vi "Field vs  IV and Ic distribution_V3.vi"() -> ()   [LabVIEW 2021]
uses:
  RT fast data.ctl
  <vilib>/LabVIEW Targets/FPGA/cRIO/shared/nicrio_ModuleControls/nicrio_cRIO-9775_RecordDataRates4ChansRing.ctl
  <vilib>/Utility/file.llb/Write Delimited Spreadsheet (DBL).vi
  Transport measurement/VIs/global.vi
  <resource>/objmgr/ni.dex.rc
  <vilib>/Analysis/NI_AALBase.lvlib
panel:
  in  "Tab Control":enum32{"Field", "cRIO", "IV Ic Parameters"}(tab)
  in  "Field Rate mT per sec":dbl=0.1 format="%#_13g"
  in  "Field Radius mT":dbl=12.0 format="%#_13g"
  in  "Field step mT":dbl=0.05 format="%#_13g"
  in  "Field Origin mT":dbl=-6.0 format="%#_13g"
  in  "Ramp up first T":bool=TRUE
  in  "Ramp type":string(combo)="Range"
  in  "Field Device Select":string(combo)="Elsa Magnet mT"
  in  "Power dbm":dbl=-135.0 format="%#_13g"
  in  "Field sub select":string(combo)="50mApV"
  in  "AI Channel":u8
  in  "Trigger Slope":enum8{"Positive", "Negative"}(ring)
  in  "Dist Record Samples":u32=10000
  in  "cRIO IP":string="//172.22.11.2"
  in  "Data buffer size":i32=1000
  in  "Voltage Scale factor":dbl=0.0001
  in  "Current Scale factor":dbl=1.0
  in  "IV Record Samples":u32=5000
  in  "Gate wait time us":u32=150
  in  "IV Record Data Rate":T1=200 items=["20.000 MS/s (NI 9775)"=1, "10.00 MS/s (NI 9775)"=2, "6.667 MS/s (NI 9775)"=3, "5.000 MS/s (NI 9775)"=4, "2.500 MS/s (NI 9775)"=8, "1.667 MS/s (NI 9775)"=12, "1.250 MS/s (NI 9775)"=16, "1.000 MS/s (NI 9775)"=20, "833.333 KS/s (NI 9775)"=24, "714.286 KS/s (NI 9775)"=28, "625.000 KS/s (NI 9775)"=32, "555.556 KS/s (NI 9775)"=36, "500.000 KS/s (NI 9775)"=40, "454.545 KS/s (NI 9775)"=44, "416.667 KS/s (NI 9775)"=48, "384.615 KS/s (NI 9775)"=52, "357.143 KS/s (NI 9775)"=56, "333.333 KS/s (NI 9775)"=60, "312.500 KS/s (NI 9775)"=64, "294.118 KS/s (NI 9775)"=68, "277.778 KS/s (NI 9775)"=72, "263.158 KS/s (NI 9775)"=76, "250.000 KS/s (NI 9775)"=80, "238.095 KS/s (NI 9775)"=84, "227.273 KS/s (NI 9775)"=88, "217.391 KS/s (NI 9775)"=92, "208.333 KS/s (NI 9775)"=96, "200.000 KS/s (NI 9775)"=100, "192.308 KS/s (NI 9775)"=104, "185.185 KS/s (NI 9775)"=108, "178.571 KS/s (NI 9775)"=112, "172.414 KS/s (NI 9775)"=116, "166.667 KS/s (NI 9775)"=120, "161.290 KS/s (NI 9775)"=124, "156.250 KS/s (NI 9775)"=128, "151.515 KS/s (NI 9775)"=132, "147.059 KS/s (NI 9775)"=136, "142.857 KS/s (NI 9775)"=140, "138.889 KS/s (NI 9775)"=144, "135.135 KS/s (NI 9775)"=148, "131.579 KS/s (NI 9775)"=152, "128.205 KS/s (NI 9775)"=156, "125.000 KS/s (NI 9775)"=160, "121.951 KS/s (NI 9775)"=164, "119.048 KS/s (NI 9775)"=168, "116.279 KS/s (NI 9775)"=172, "113.636 KS/s (NI 9775)"=176, "111.111 KS/s (NI 9775)"=180, "108.696 KS/s (NI 9775)"=184, "106.383 KS/s (NI 9775)"=188, "104.167 KS/s (NI 9775)"=192, "102.041 KS/s (NI 9775)"=196, "100.000 KS/s (NI 9775)"=200, "50.000 KS/s (NI 9775)"=400, "33.333 KS/s (NI 9775)"=600, "25.000 KS/s (NI 9775)"=800, "20.000 KS/s (NI 9775)"=1000, "16.667 KS/s (NI 9775)"=1200, "14.286 KS/s (NI 9775)"=1400, "12.500 KS/s (NI 9775)"=1600, "11.111 KS/s (NI 9775)"=1800, "10.000 KS/s (NI 9775)"=2000, "9.091 KS/s (NI 9775)"=2200, "8.333 KS/s (NI 9775)"=2400, "7.692 KS/s (NI 9775)"=2600, "7.143 KS/s (NI 9775)"=2800, "6.667 KS/s (NI 9775)"=3000, "6.250 KS/s (NI 9775)"=3200, "5.882 KS/s (NI 9775)"=3400, "5.556 KS/s (NI 9775)"=3600, "5.000 KS/s (NI 9775)"=4000, "4.762 KS/s (NI 9775)"=4200, "4.545 KS/s (NI 9775)"=4400, "4.348 KS/s (NI 9775)"=4600, "4.167 KS/s (NI 9775)"=4800, "4.000 KS/s (NI 9775)"=5000, "3.846 KS/s (NI 9775)"=5200, "3.571 KS/s (NI 9775)"=5600, "3.333 KS/s (NI 9775)"=6000, "3.125 KS/s (NI 9775)"=6400, "2.941 KS/s (NI 9775)"=6800, "2.778 KS/s (NI 9775)"=7200, "2.632 KS/s (NI 9775)"=7600, "2.500 KS/s (NI 9775)"=8000, "2.381 KS/s (NI 9775)"=8400, "2.273 KS/s (NI 9775)"=8800, "2.174 KS/s (NI 9775)"=9200, "2.083 KS/s (NI 9775)"=9600, "2.000 KS/s (NI 9775)"=10000, "1.923 KS/s (NI 9775)"=10400, "1.852 KS/s (NI 9775)"=10800, "1.786 KS/s (NI 9775)"=11200, "1.724 KS/s (NI 9775)"=11600, "1.667 KS/s (NI 9775)"=12000, "1.613 KS/s (NI 9775)"=12400, "1.563 KS/s (NI 9775)"=12800, "1.515 KS/s (NI 9775)"=13200, "1.471 KS/s (NI 9775)"=13600, "1.429 KS/s (NI 9775)"=14000, "1.389 KS/s (NI 9775)"=14400, "1.351 KS/s (NI 9775)"=14800, "1.316 KS/s (NI 9775)"=15200, "1.282 KS/s (NI 9775)"=15600, "1.250 KS/s (NI 9775)"=16000, "1.220 KS/s (NI 9775)"=16400, "1.190 KS/s (NI 9775)"=16800, "1.163 KS/s (NI 9775)"=17200, "1.136 KS/s (NI 9775)"=17600, "1.111 KS/s (NI 9775)"=18000, "1.087 KS/s (NI 9775)"=18400, "1.064 KS/s (NI 9775)"=18800, "1.042 KS/s (NI 9775)"=19200, "1.020 KS/s (NI 9775)"=19600, "1.000 KS/s (NI 9775)"=20000, "0.980 KS/s (NI 9775)"=20400, "0.962 KS/s (NI 9775)"=20800, "0.943 KS/s (NI 9775)"=21200, "0.926 KS/s (NI 9775)"=21600, "0.909 KS/s (NI 9775)"=22000, "0.893 KS/s (NI 9775)"=22400, "0.877 KS/s (NI 9775)"=22800, "0.862 KS/s (NI 9775)"=23200, "0.847 KS/s (NI 9775)"=23600, "0.833 KS/s (NI 9775)"=24000, "0.820 KS/s (NI 9775)"=24400, "0.806 KS/s (NI 9775)"=24800, "0.794 KS/s (NI 9775)"=25200, "0.781 KS/s (NI 9775)"=25600, "0.694 KS/s (NI 9775)"=28800, "0.625 KS/s (NI 9775)"=32000, "0.568 KS/s (NI 9775)"=35200, "0.521 KS/s (NI 9775)"=38400, "0.446 KS/s (NI 9775)"=44800, "0.391 KS/s (NI 9775)"=51200, "0.347 KS/s (NI 9775)"=57600, "0.313 KS/s (NI 9775)"=64000]
  in  "Relative threshold":dbl=0.25 format="%#_13g"
  in  "Dist Record Data Rate":T1=1 items=["20.000 MS/s (NI 9775)"=1, "10.00 MS/s (NI 9775)"=2, "6.667 MS/s (NI 9775)"=3, "5.000 MS/s (NI 9775)"=4, "2.500 MS/s (NI 9775)"=8, "1.667 MS/s (NI 9775)"=12, "1.250 MS/s (NI 9775)"=16, "1.000 MS/s (NI 9775)"=20, "833.333 KS/s (NI 9775)"=24, "714.286 KS/s (NI 9775)"=28, "625.000 KS/s (NI 9775)"=32, "555.556 KS/s (NI 9775)"=36, "500.000 KS/s (NI 9775)"=40, "454.545 KS/s (NI 9775)"=44, "416.667 KS/s (NI 9775)"=48, "384.615 KS/s (NI 9775)"=52, "357.143 KS/s (NI 9775)"=56, "333.333 KS/s (NI 9775)"=60, "312.500 KS/s (NI 9775)"=64, "294.118 KS/s (NI 9775)"=68, "277.778 KS/s (NI 9775)"=72, "263.158 KS/s (NI 9775)"=76, "250.000 KS/s (NI 9775)"=80, "238.095 KS/s (NI 9775)"=84, "227.273 KS/s (NI 9775)"=88, "217.391 KS/s (NI 9775)"=92, "208.333 KS/s (NI 9775)"=96, "200.000 KS/s (NI 9775)"=100, "192.308 KS/s (NI 9775)"=104, "185.185 KS/s (NI 9775)"=108, "178.571 KS/s (NI 9775)"=112, "172.414 KS/s (NI 9775)"=116, "166.667 KS/s (NI 9775)"=120, "161.290 KS/s (NI 9775)"=124, "156.250 KS/s (NI 9775)"=128, "151.515 KS/s (NI 9775)"=132, "147.059 KS/s (NI 9775)"=136, "142.857 KS/s (NI 9775)"=140, "138.889 KS/s (NI 9775)"=144, "135.135 KS/s (NI 9775)"=148, "131.579 KS/s (NI 9775)"=152, "128.205 KS/s (NI 9775)"=156, "125.000 KS/s (NI 9775)"=160, "121.951 KS/s (NI 9775)"=164, "119.048 KS/s (NI 9775)"=168, "116.279 KS/s (NI 9775)"=172, "113.636 KS/s (NI 9775)"=176, "111.111 KS/s (NI 9775)"=180, "108.696 KS/s (NI 9775)"=184, "106.383 KS/s (NI 9775)"=188, "104.167 KS/s (NI 9775)"=192, "102.041 KS/s (NI 9775)"=196, "100.000 KS/s (NI 9775)"=200, "50.000 KS/s (NI 9775)"=400, "33.333 KS/s (NI 9775)"=600, "25.000 KS/s (NI 9775)"=800, "20.000 KS/s (NI 9775)"=1000, "16.667 KS/s (NI 9775)"=1200, "14.286 KS/s (NI 9775)"=1400, "12.500 KS/s (NI 9775)"=1600, "11.111 KS/s (NI 9775)"=1800, "10.000 KS/s (NI 9775)"=2000, "9.091 KS/s (NI 9775)"=2200, "8.333 KS/s (NI 9775)"=2400, "7.692 KS/s (NI 9775)"=2600, "7.143 KS/s (NI 9775)"=2800, "6.667 KS/s (NI 9775)"=3000, "6.250 KS/s (NI 9775)"=3200, "5.882 KS/s (NI 9775)"=3400, "5.556 KS/s (NI 9775)"=3600, "5.000 KS/s (NI 9775)"=4000, "4.762 KS/s (NI 9775)"=4200, "4.545 KS/s (NI 9775)"=4400, "4.348 KS/s (NI 9775)"=4600, "4.167 KS/s (NI 9775)"=4800, "4.000 KS/s (NI 9775)"=5000, "3.846 KS/s (NI 9775)"=5200, "3.571 KS/s (NI 9775)"=5600, "3.333 KS/s (NI 9775)"=6000, "3.125 KS/s (NI 9775)"=6400, "2.941 KS/s (NI 9775)"=6800, "2.778 KS/s (NI 9775)"=7200, "2.632 KS/s (NI 9775)"=7600, "2.500 KS/s (NI 9775)"=8000, "2.381 KS/s (NI 9775)"=8400, "2.273 KS/s (NI 9775)"=8800, "2.174 KS/s (NI 9775)"=9200, "2.083 KS/s (NI 9775)"=9600, "2.000 KS/s (NI 9775)"=10000, "1.923 KS/s (NI 9775)"=10400, "1.852 KS/s (NI 9775)"=10800, "1.786 KS/s (NI 9775)"=11200, "1.724 KS/s (NI 9775)"=11600, "1.667 KS/s (NI 9775)"=12000, "1.613 KS/s (NI 9775)"=12400, "1.563 KS/s (NI 9775)"=12800, "1.515 KS/s (NI 9775)"=13200, "1.471 KS/s (NI 9775)"=13600, "1.429 KS/s (NI 9775)"=14000, "1.389 KS/s (NI 9775)"=14400, "1.351 KS/s (NI 9775)"=14800, "1.316 KS/s (NI 9775)"=15200, "1.282 KS/s (NI 9775)"=15600, "1.250 KS/s (NI 9775)"=16000, "1.220 KS/s (NI 9775)"=16400, "1.190 KS/s (NI 9775)"=16800, "1.163 KS/s (NI 9775)"=17200, "1.136 KS/s (NI 9775)"=17600, "1.111 KS/s (NI 9775)"=18000, "1.087 KS/s (NI 9775)"=18400, "1.064 KS/s (NI 9775)"=18800, "1.042 KS/s (NI 9775)"=19200, "1.020 KS/s (NI 9775)"=19600, "1.000 KS/s (NI 9775)"=20000, "0.980 KS/s (NI 9775)"=20400, "0.962 KS/s (NI 9775)"=20800, "0.943 KS/s (NI 9775)"=21200, "0.926 KS/s (NI 9775)"=21600, "0.909 KS/s (NI 9775)"=22000, "0.893 KS/s (NI 9775)"=22400, "0.877 KS/s (NI 9775)"=22800, "0.862 KS/s (NI 9775)"=23200, "0.847 KS/s (NI 9775)"=23600, "0.833 KS/s (NI 9775)"=24000, "0.820 KS/s (NI 9775)"=24400, "0.806 KS/s (NI 9775)"=24800, "0.794 KS/s (NI 9775)"=25200, "0.781 KS/s (NI 9775)"=25600, "0.694 KS/s (NI 9775)"=28800, "0.625 KS/s (NI 9775)"=32000, "0.568 KS/s (NI 9775)"=35200, "0.521 KS/s (NI 9775)"=38400, "0.446 KS/s (NI 9775)"=44800, "0.391 KS/s (NI 9775)"=51200, "0.347 KS/s (NI 9775)"=57600, "0.313 KS/s (NI 9775)"=64000]
  in  "Zero avg":i32=500
  in  "Count us half of T":u32=1
  in  "Wait before trigger us":u32=10100
  in  "Tab Control 2":enum32{"IV", "Ic"}(tab)
  out "IV parameters":T2={"Records Num"=1, "AI Trigger Configuration"={"Trigger Slope"=enum."Positive", "Trigger Level"=0.10009765625, "Hystesis Value"=0.094970703125, "AI Channel"=0}, "Record PreTrigger Samples"=1, "Record Samples"=5000, "Ic Cut off or curve"=FALSE, "Gate wait time us"=150, "Record Data Rate"=200, "Count us half of T"=1, "Wait before trigger us"=10100, "Cutoff delay usec"=0} {"Record Data Rate" items=["20.000 MS/s (NI 9775)"=1, "10.00 MS/s (NI 9775)"=2, "6.667 MS/s (NI 9775)"=3, "5.000 MS/s (NI 9775)"=4, "2.500 MS/s (NI 9775)"=8, "1.667 MS/s (NI 9775)"=12, "1.250 MS/s (NI 9775)"=16, "1.000 MS/s (NI 9775)"=20, "833.333 KS/s (NI 9775)"=24, "714.286 KS/s (NI 9775)"=28, "625.000 KS/s (NI 9775)"=32, "555.556 KS/s (NI 9775)"=36, "500.000 KS/s (NI 9775)"=40, "454.545 KS/s (NI 9775)"=44, "416.667 KS/s (NI 9775)"=48, "384.615 KS/s (NI 9775)"=52, "357.143 KS/s (NI 9775)"=56, "333.333 KS/s (NI 9775)"=60, "312.500 KS/s (NI 9775)"=64, "294.118 KS/s (NI 9775)"=68, "277.778 KS/s (NI 9775)"=72, "263.158 KS/s (NI 9775)"=76, "250.000 KS/s (NI 9775)"=80, "238.095 KS/s (NI 9775)"=84, "227.273 KS/s (NI 9775)"=88, "217.391 KS/s (NI 9775)"=92, "208.333 KS/s (NI 9775)"=96, "200.000 KS/s (NI 9775)"=100, "192.308 KS/s (NI 9775)"=104, "185.185 KS/s (NI 9775)"=108, "178.571 KS/s (NI 9775)"=112, "172.414 KS/s (NI 9775)"=116, "166.667 KS/s (NI 9775)"=120, "161.290 KS/s (NI 9775)"=124, "156.250 KS/s (NI 9775)"=128, "151.515 KS/s (NI 9775)"=132, "147.059 KS/s (NI 9775)"=136, "142.857 KS/s (NI 9775)"=140, "138.889 KS/s (NI 9775)"=144, "135.135 KS/s (NI 9775)"=148, "131.579 KS/s (NI 9775)"=152, "128.205 KS/s (NI 9775)"=156, "125.000 KS/s (NI 9775)"=160, "121.951 KS/s (NI 9775)"=164, "119.048 KS/s (NI 9775)"=168, "116.279 KS/s (NI 9775)"=172, "113.636 KS/s (NI 9775)"=176, "111.111 KS/s (NI 9775)"=180, "108.696 KS/s (NI 9775)"=184, "106.383 KS/s (NI 9775)"=188, "104.167 KS/s (NI 9775)"=192, "102.041 KS/s (NI 9775)"=196, "100.000 KS/s (NI 9775)"=200, "50.000 KS/s (NI 9775)"=400, "33.333 KS/s (NI 9775)"=600, "25.000 KS/s (NI 9775)"=800, "20.000 KS/s (NI 9775)"=1000, "16.667 KS/s (NI 9775)"=1200, "14.286 KS/s (NI 9775)"=1400, "12.500 KS/s (NI 9775)"=1600, "11.111 KS/s (NI 9775)"=1800, "10.000 KS/s (NI 9775)"=2000, "9.091 KS/s (NI 9775)"=2200, "8.333 KS/s (NI 9775)"=2400, "7.692 KS/s (NI 9775)"=2600, "7.143 KS/s (NI 9775)"=2800, "6.667 KS/s (NI 9775)"=3000, "6.250 KS/s (NI 9775)"=3200, "5.882 KS/s (NI 9775)"=3400, "5.556 KS/s (NI 9775)"=3600, "5.000 KS/s (NI 9775)"=4000, "4.762 KS/s (NI 9775)"=4200, "4.545 KS/s (NI 9775)"=4400, "4.348 KS/s (NI 9775)"=4600, "4.167 KS/s (NI 9775)"=4800, "4.000 KS/s (NI 9775)"=5000, "3.846 KS/s (NI 9775)"=5200, "3.571 KS/s (NI 9775)"=5600, "3.333 KS/s (NI 9775)"=6000, "3.125 KS/s (NI 9775)"=6400, "2.941 KS/s (NI 9775)"=6800, "2.778 KS/s (NI 9775)"=7200, "2.632 KS/s (NI 9775)"=7600, "2.500 KS/s (NI 9775)"=8000, "2.381 KS/s (NI 9775)"=8400, "2.273 KS/s (NI 9775)"=8800, "2.174 KS/s (NI 9775)"=9200, "2.083 KS/s (NI 9775)"=9600, "2.000 KS/s (NI 9775)"=10000, "1.923 KS/s (NI 9775)"=10400, "1.852 KS/s (NI 9775)"=10800, "1.786 KS/s (NI 9775)"=11200, "1.724 KS/s (NI 9775)"=11600, "1.667 KS/s (NI 9775)"=12000, "1.613 KS/s (NI 9775)"=12400, "1.563 KS/s (NI 9775)"=12800, "1.515 KS/s (NI 9775)"=13200, "1.471 KS/s (NI 9775)"=13600, "1.429 KS/s (NI 9775)"=14000, "1.389 KS/s (NI 9775)"=14400, "1.351 KS/s (NI 9775)"=14800, "1.316 KS/s (NI 9775)"=15200, "1.282 KS/s (NI 9775)"=15600, "1.250 KS/s (NI 9775)"=16000, "1.220 KS/s (NI 9775)"=16400, "1.190 KS/s (NI 9775)"=16800, "1.163 KS/s (NI 9775)"=17200, "1.136 KS/s (NI 9775)"=17600, "1.111 KS/s (NI 9775)"=18000, "1.087 KS/s (NI 9775)"=18400, "1.064 KS/s (NI 9775)"=18800, "1.042 KS/s (NI 9775)"=19200, "1.020 KS/s (NI 9775)"=19600, "1.000 KS/s (NI 9775)"=20000, "0.980 KS/s (NI 9775)"=20400, "0.962 KS/s (NI 9775)"=20800, "0.943 KS/s (NI 9775)"=21200, "0.926 KS/s (NI 9775)"=21600, "0.909 KS/s (NI 9775)"=22000, "0.893 KS/s (NI 9775)"=22400, "0.877 KS/s (NI 9775)"=22800, "0.862 KS/s (NI 9775)"=23200, "0.847 KS/s (NI 9775)"=23600, "0.833 KS/s (NI 9775)"=24000, "0.820 KS/s (NI 9775)"=24400, "0.806 KS/s (NI 9775)"=24800, "0.794 KS/s (NI 9775)"=25200, "0.781 KS/s (NI 9775)"=25600, "0.694 KS/s (NI 9775)"=28800, "0.625 KS/s (NI 9775)"=32000, "0.568 KS/s (NI 9775)"=35200, "0.521 KS/s (NI 9775)"=38400, "0.446 KS/s (NI 9775)"=44800, "0.391 KS/s (NI 9775)"=51200, "0.347 KS/s (NI 9775)"=57600, "0.313 KS/s (NI 9775)"=64000]}
  out "Ic parameters":T2={"Records Num"=10000, "AI Trigger Configuration"={"Trigger Slope"=enum."Positive", "Trigger Level"=0.267822265625, "Hystesis Value"=0.0, "AI Channel"=0}, "Record PreTrigger Samples"=1, "Record Samples"=16, "Ic Cut off or curve"=TRUE, "Gate wait time us"=150, "Record Data Rate"=1, "Count us half of T"=1, "Wait before trigger us"=10100, "Cutoff delay usec"=0} {"Record Data Rate" items=["20.000 MS/s (NI 9775)"=1, "10.00 MS/s (NI 9775)"=2, "6.667 MS/s (NI 9775)"=3, "5.000 MS/s (NI 9775)"=4, "2.500 MS/s (NI 9775)"=8, "1.667 MS/s (NI 9775)"=12, "1.250 MS/s (NI 9775)"=16, "1.000 MS/s (NI 9775)"=20, "833.333 KS/s (NI 9775)"=24, "714.286 KS/s (NI 9775)"=28, "625.000 KS/s (NI 9775)"=32, "555.556 KS/s (NI 9775)"=36, "500.000 KS/s (NI 9775)"=40, "454.545 KS/s (NI 9775)"=44, "416.667 KS/s (NI 9775)"=48, "384.615 KS/s (NI 9775)"=52, "357.143 KS/s (NI 9775)"=56, "333.333 KS/s (NI 9775)"=60, "312.500 KS/s (NI 9775)"=64, "294.118 KS/s (NI 9775)"=68, "277.778 KS/s (NI 9775)"=72, "263.158 KS/s (NI 9775)"=76, "250.000 KS/s (NI 9775)"=80, "238.095 KS/s (NI 9775)"=84, "227.273 KS/s (NI 9775)"=88, "217.391 KS/s (NI 9775)"=92, "208.333 KS/s (NI 9775)"=96, "200.000 KS/s (NI 9775)"=100, "192.308 KS/s (NI 9775)"=104, "185.185 KS/s (NI 9775)"=108, "178.571 KS/s (NI 9775)"=112, "172.414 KS/s (NI 9775)"=116, "166.667 KS/s (NI 9775)"=120, "161.290 KS/s (NI 9775)"=124, "156.250 KS/s (NI 9775)"=128, "151.515 KS/s (NI 9775)"=132, "147.059 KS/s (NI 9775)"=136, "142.857 KS/s (NI 9775)"=140, "138.889 KS/s (NI 9775)"=144, "135.135 KS/s (NI 9775)"=148, "131.579 KS/s (NI 9775)"=152, "128.205 KS/s (NI 9775)"=156, "125.000 KS/s (NI 9775)"=160, "121.951 KS/s (NI 9775)"=164, "119.048 KS/s (NI 9775)"=168, "116.279 KS/s (NI 9775)"=172, "113.636 KS/s (NI 9775)"=176, "111.111 KS/s (NI 9775)"=180, "108.696 KS/s (NI 9775)"=184, "106.383 KS/s (NI 9775)"=188, "104.167 KS/s (NI 9775)"=192, "102.041 KS/s (NI 9775)"=196, "100.000 KS/s (NI 9775)"=200, "50.000 KS/s (NI 9775)"=400, "33.333 KS/s (NI 9775)"=600, "25.000 KS/s (NI 9775)"=800, "20.000 KS/s (NI 9775)"=1000, "16.667 KS/s (NI 9775)"=1200, "14.286 KS/s (NI 9775)"=1400, "12.500 KS/s (NI 9775)"=1600, "11.111 KS/s (NI 9775)"=1800, "10.000 KS/s (NI 9775)"=2000, "9.091 KS/s (NI 9775)"=2200, "8.333 KS/s (NI 9775)"=2400, "7.692 KS/s (NI 9775)"=2600, "7.143 KS/s (NI 9775)"=2800, "6.667 KS/s (NI 9775)"=3000, "6.250 KS/s (NI 9775)"=3200, "5.882 KS/s (NI 9775)"=3400, "5.556 KS/s (NI 9775)"=3600, "5.000 KS/s (NI 9775)"=4000, "4.762 KS/s (NI 9775)"=4200, "4.545 KS/s (NI 9775)"=4400, "4.348 KS/s (NI 9775)"=4600, "4.167 KS/s (NI 9775)"=4800, "4.000 KS/s (NI 9775)"=5000, "3.846 KS/s (NI 9775)"=5200, "3.571 KS/s (NI 9775)"=5600, "3.333 KS/s (NI 9775)"=6000, "3.125 KS/s (NI 9775)"=6400, "2.941 KS/s (NI 9775)"=6800, "2.778 KS/s (NI 9775)"=7200, "2.632 KS/s (NI 9775)"=7600, "2.500 KS/s (NI 9775)"=8000, "2.381 KS/s (NI 9775)"=8400, "2.273 KS/s (NI 9775)"=8800, "2.174 KS/s (NI 9775)"=9200, "2.083 KS/s (NI 9775)"=9600, "2.000 KS/s (NI 9775)"=10000, "1.923 KS/s (NI 9775)"=10400, "1.852 KS/s (NI 9775)"=10800, "1.786 KS/s (NI 9775)"=11200, "1.724 KS/s (NI 9775)"=11600, "1.667 KS/s (NI 9775)"=12000, "1.613 KS/s (NI 9775)"=12400, "1.563 KS/s (NI 9775)"=12800, "1.515 KS/s (NI 9775)"=13200, "1.471 KS/s (NI 9775)"=13600, "1.429 KS/s (NI 9775)"=14000, "1.389 KS/s (NI 9775)"=14400, "1.351 KS/s (NI 9775)"=14800, "1.316 KS/s (NI 9775)"=15200, "1.282 KS/s (NI 9775)"=15600, "1.250 KS/s (NI 9775)"=16000, "1.220 KS/s (NI 9775)"=16400, "1.190 KS/s (NI 9775)"=16800, "1.163 KS/s (NI 9775)"=17200, "1.136 KS/s (NI 9775)"=17600, "1.111 KS/s (NI 9775)"=18000, "1.087 KS/s (NI 9775)"=18400, "1.064 KS/s (NI 9775)"=18800, "1.042 KS/s (NI 9775)"=19200, "1.020 KS/s (NI 9775)"=19600, "1.000 KS/s (NI 9775)"=20000, "0.980 KS/s (NI 9775)"=20400, "0.962 KS/s (NI 9775)"=20800, "0.943 KS/s (NI 9775)"=21200, "0.926 KS/s (NI 9775)"=21600, "0.909 KS/s (NI 9775)"=22000, "0.893 KS/s (NI 9775)"=22400, "0.877 KS/s (NI 9775)"=22800, "0.862 KS/s (NI 9775)"=23200, "0.847 KS/s (NI 9775)"=23600, "0.833 KS/s (NI 9775)"=24000, "0.820 KS/s (NI 9775)"=24400, "0.806 KS/s (NI 9775)"=24800, "0.794 KS/s (NI 9775)"=25200, "0.781 KS/s (NI 9775)"=25600, "0.694 KS/s (NI 9775)"=28800, "0.625 KS/s (NI 9775)"=32000, "0.568 KS/s (NI 9775)"=35200, "0.521 KS/s (NI 9775)"=38400, "0.446 KS/s (NI 9775)"=44800, "0.391 KS/s (NI 9775)"=51200, "0.347 KS/s (NI 9775)"=57600, "0.313 KS/s (NI 9775)"=64000]}
  out "Threshold":dbl=0.26789404296875
  in  "Stop loop":bool
  out "Current Field mT":dbl=6.0
  in  "Name":string="book791"
  in  "Contour plot folder":path=path "C:/Users/gyue/Desktop/20221209 G22L measurement"
  out "Histogram Graph":T3(graph)={"X Values"=[0.174517822265625, 0.177850341796875, 0.181182861328125, 0.184515380859375, 0.187847900390625, 0.19118041992187498, 0.19451293945312498, 0.19784545898437497, 0.20117797851562497, 0.20451049804687496, 0.20784301757812496, 0.21117553710937495, 0.21450805664062494, 0.21784057617187494, 0.22117309570312493, 0.22450561523437493, 0.22783813476562492, 0.23117065429687492, 0.2345031738281249, 0.2378356933593749, 0.2411682128906249, 0.2445007324218749, 0.2478332519531249, 0.2511657714843749, 0.25449829101562493, 0.25783081054687496, 0.261163330078125, 0.264495849609375, 0.267828369140625, 0.27116088867187504, 0.27449340820312507, 0.2778259277343751, 0.2811584472656251, 0.28449096679687513, 0.28782348632812516, 0.2911560058593752, 0.2944885253906252, 0.2978210449218752, 0.30115356445312524, 0.30448608398437527, 0.3078186035156253, 0.3111511230468753, 0.31448364257812533, 0.31781616210937536, 0.3211486816406254, 0.3244812011718754, 0.3278137207031254, 0.33114624023437544, 0.33447875976562547, 0.3378112792968755, 0.3411437988281255, 0.34447631835937553, 0.34780883789062556, 0.3511413574218756, 0.3544738769531256, 0.3578063964843756, 0.36113891601562564, 0.36447143554687567, 0.3678039550781257, 0.3711364746093757, 0.37446899414062573, 0.37780151367187575, 0.3811340332031258, 0.3844665527343758, 0.3877990722656258, 0.39113159179687584, 0.39446411132812587, 0.3977966308593759, 0.4011291503906259, 0.40446166992187593, 0.40779418945312595, 0.411126708984376, 0.414459228515626, 0.417791748046876, 0.42112426757812604, 0.42445678710937607, 0.4277893066406261, 0.4311218261718761, 0.43445434570312613, 0.43778686523437615, 0.4411193847656262, 0.4444519042968762, 0.4477844238281262, 0.45111694335937624, 0.45444946289062627, 0.4577819824218763, 0.4611145019531263, 0.46444702148437633, 0.46777954101562635, 0.4711120605468764, 0.4744445800781264, 0.4777770996093764, 0.48110961914062644, 0.48444213867187647, 0.4877746582031265, 0.4911071777343765, 0.49443969726562653, 0.49777221679687655, 0.5011047363281266, 0.5044372558593766], "Histogram: h(x)"=[1, 0, 0, 0, 1, 0, 0, 0, 0, 0, 0, 0, 0, 0, 1, 0, 0, 0, 1, 1, 0, 1, 3, 0, 0, 0, 1, 0, 1, 3, 0, 1, 1, 2, 0, 1, 1, 0, 4, 3, 2, 5, 2, 10, 4, 5, 8, 14, 23, 11, 25, 34, 25, 56, 44, 54, 112, 95, 182, 122, 230, 169, 189, 365, 268, 427, 341, 333, 599, 397, 620, 440, 378, 664, 365, 557, 356, 320, 470, 252, 349, 206, 148, 195, 99, 126, 67, 61, 34, 26, 28, 16, 15, 9, 7, 9, 1, 2, 0, 2]}
  out "IV curve":cluster{"Y":dbl[], "Y":dbl[]}[](graph)
  out "error out":errorcluster
  # "unit is dBm GHz for RF"
  # "Voltage x factor=uA"
  # "Voltage x factor=V"
  # "IV setting"
  # "Distribution setting"
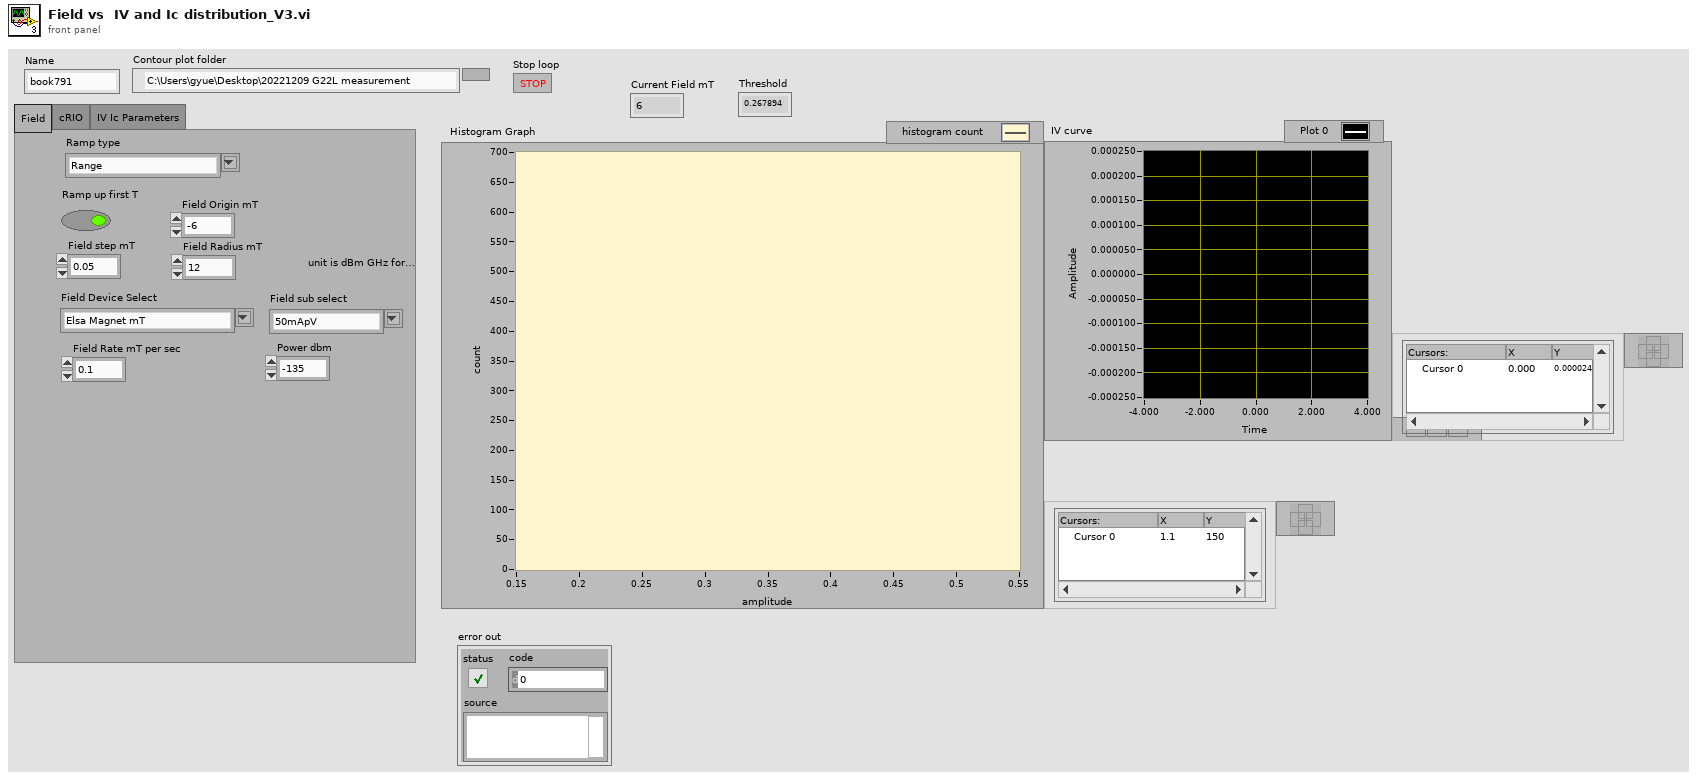
[diagram p1: front panel]
types:
  T1 = typedef "nicrio_cRIO-9775_RecordDataRates4ChansRing.ctl" = u16
  T2 = typedef "RT fast data.ctl" = cluster{"Records Num":i32, "AI Trigger Configuration":cluster{"Trigger Slope":enum8{"Positive", "Negative"}, "Trigger Level":fxp<+/-,17,5>, "Hystesis Value":fxp<+,16,4>, "AI Channel":u8}, "Record PreTrigger Samples":u32, "Record Samples":u32, "Ic Cut off or curve":bool, "Gate wait time us":u32, "Record Data Rate":T1, "Count us half of T":u32, "Wait before trigger us":u32, "Cutoff delay usec":u32}
  T3 = cluster{"X Values":dbl[], "Histogram: h(x)":i32[]}
  T4 = cluster{"Trigger Slope":enum8{"Positive", "Negative"}, "Trigger Level":fxp<+/-,17,5>, "Hystesis Value":fxp<+,16,4>, "AI Channel":u8}
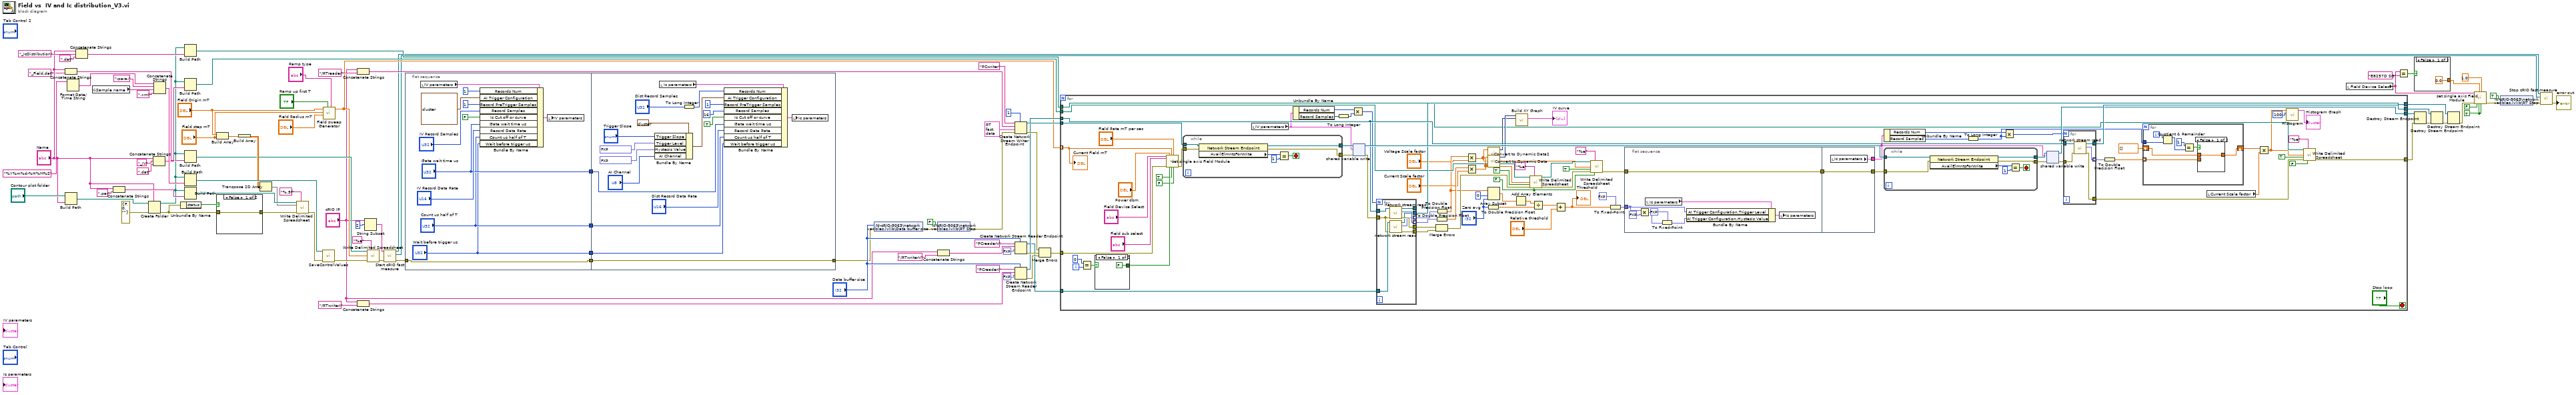
[diagram p0: block diagram]
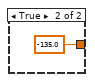
[diagram p2: hidden frame]
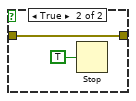
[diagram p3: hidden frame]
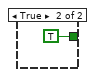
[diagram p4: hidden frame]
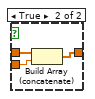
[diagram p5: hidden frame]
diagram:
  w19 = TRUE ("final")
  n1 = Concatenate Strings("Name", "_Field.dat" ("string")) -> (w34:string)
  n2 = Build Path(base path="Contour plot folder", name or relative path="Name") -> (appended path=w52:path)
  n3 = Format Date/Time String(time format string (%c)="%Y%m%d-%H%M%S") -> (date/time string=w48:string)  [unwired: 2 in]
  n4 = Concatenate Strings("Name", "_IcDistribution" ("string"), ".dat" ("string")) -> (w41:string)
  n5 = global read "global.vi" "Sample name"() -> (w47:string)
  n6 = Concatenate Strings("Name", ".par" ("string")) -> (w59:string)
  n7 = Create Folder(prompt (Create Folder)="Name", path (use dialog)=w52, error in=errorcluster {"status"=FALSE, "code"=0, "source"=""}) -> (created path=w33:path, error out=w49:errorcluster)  [unwired: 1 out]
  n8 = Concatenate Strings("Name", "_IV" ("string"), ".dat" ("string")) -> (w53:string)
  n9 = Concatenate Strings(w48, "-para-" ("string"), w47, ".xml" ("string")) -> (w63:string)
  n10 = Unbundle By Name(w49) -> ("status"=w50:bool)
  n11 = Build Path(base path=w33, name or relative path=w41) -> (appended path=w39:path)
  n12 = Build Path(base path=w33, name or relative path=w53) -> (appended path=w40:path)
  n13 = Build Path(base path=w33, name or relative path=w34) -> (appended path=w32:path)
  n14 = Build Path(base path=w33, name or relative path=w63) -> (appended path=w61:path)
  n15 = Build Path(base path=w33, name or relative path=w59) -> (appended path=w58:path)
  n16 = Build Array("Field Origin mT", "Field step mT") -> (w56:dbl[])
  n17 = case shown="False" w50 {
    tunnel: [w97 w99] -> w3
    tunnel: w49 -> [w97 w99]
    frame False {
    }
    frame True {
      n18 = Stop(stop? (T)=TRUE) -> ()
    }
  }
  n19 = Build Array(w56) -> (w55:dbl[][])
  n20 = Transpose 2D Array(2D array=w55) -> (transposed array=w54:dbl[][])
  n21 = call-poly <vilib>:"Write Delimited Spreadsheet.vi"("file path (dialog if empty)"=w58, "format (%.3f)"="%.5f", "2D data"=w54, "error in (no error)"=w3) -> ("error out"=w51:errorcluster)  [unwired: 10 in, 1 out]
  n22 = call "SaveControlValues.vi"("XML File Path"=w61, "error in (no error)"=w51) -> ("error out"=w30:errorcluster)  [unwired: 8 in]
  n23 = call "Field sweep Generator.vi"("Ramp type"="Ramp type", "Ramp up first T"="Ramp up first T", "Field Radius"="Field Radius mT", "Field step"="Field step mT", "Field Origin"="Field Origin mT") -> ("output array"=w26:dbl[])  [unwired: 6 in]
  n24 = Concatenate Strings("cRIO IP", "/RTreader" ("string")) -> (w92:string)
  n25 = Concatenate Strings("cRIO IP", "/RTwriterI" ("string")) -> (w78:string)
  n26 = String Subset(string="cRIO IP", offset (0)=2) -> (substring=w4:string)  [unwired: 1 in]
  n27 = call-poly <vilib>:"Write Delimited Spreadsheet.vi"("file path (dialog if empty)"=w32, "format (%.3f)"="%e", "1D data"=w26, "error in (no error)"=w30) -> ("error out"=w2:errorcluster)  [unwired: 10 in, 1 out]
  n28 = call "Start cRIO fast measure.vi"("error in (no error)"=w2, "machine IP"=w4) -> ("error out"=w1:errorcluster, "vi reference"=w13:refnum<vi>, "application reference"=w14:refnum<vi>)  [unwired: 7 in]
  n29 = flat-sequence {
    tunnel: w1 -> [w111]
    tunnel: [w111] -> w28
    tunnel: ["Gate wait time us"] -> w27
    tunnel: ["Count us half of T"] -> w16
    tunnel: ["Wait before trigger us"] -> w15
    tunnel: [w129] -> w29
    tunnel: w28 -> [w129]
    tunnel: w27 -> [w121]
    tunnel: w16 -> [w113]
    tunnel: w15 -> [w112]
    frame #0 {
      n30 = local read "IV parameters"() -> (w110:T2)
      n31 = Bundle By Name(cluster=w110, "Records Num"=1, "AI Trigger Configuration"=T4 {"Trigger Slope"=enum."Positive", "Trigger Level"=0.10009765625, "Hystesis Value"=0.094970703125, "AI Channel"=0}, "Record PreTrigger Samples"=u32 1, "Record Samples"="IV Record Samples", "Ic Cut off or curve"=FALSE, "Gate wait time us"="Gate wait time us", "Record Data Rate"="IV Record Data Rate", "Count us half of T"="Count us half of T", "Wait before trigger us"="Wait before trigger us") -> (w102:T2)
      n32 = local write "IV parameters"(w102) -> ()
    }
    frame #1 {
      n33 = Bundle By Name(cluster=T4 {"Trigger Slope"=enum."Positive", "Trigger Level"=0.1708984375, "Hystesis Value"=0.162353515625, "AI Channel"=0} ("AI Trigger Configuration"), "Trigger Slope"="Trigger Slope", "Trigger Level"=fxp<+/-,17,5> 0.14990234375, "Hystesis Value"=fxp<+,16,4> 0.10009765625, "AI Channel"="AI Channel") -> (w117:T4)
      n34 = local read "Ic parameters"() -> (w128:T2)
      n35 = To Long Integer(number="Dist Record Samples") -> (32bit integer=w126:i32)
      n36 = Bundle By Name(cluster=w128, "Records Num"=w126, "AI Trigger Configuration"=w117, "Record PreTrigger Samples"=u32 1, "Record Samples"=u32 16, "Ic Cut off or curve"=TRUE, "Gate wait time us"=w121, "Record Data Rate"="Dist Record Data Rate", "Count us half of T"=w113, "Wait before trigger us"=w112) -> (w116:T2)
      n37 = local write "Ic parameters"(w116) -> ()
    }
  }
  n38 = shared-variable "NI-cRIO-9063\\network varibles.lvlib\\Data buffer size"("Data buffer size", error in=w29) -> (error out=w76:errorcluster)
  n39 = shared-variable "NI-cRIO-9063\\network varibles.lvlib\\RT Stop"(FALSE ("RT Stop"), error in=w76) -> (error out=w83:errorcluster)
  n40 = Concatenate Strings("cRIO IP", "/RTwriterV" ("string")) -> (w85:string)
  n41 = Create Network Stream Writer Endpoint(7:1 ("writer buffer size"), 8:w83, 9:T2 {"Records Num"=0, "AI Trigger Configuration"={"Trigger Slope"=enum."Positive", "Trigger Level"=0.0, "Hystesis Value"=0.0, "AI Channel"=0}, "Record PreTrigger Samples"=0, "Record Samples"=0, "Ic Cut off or curve"=FALSE, "Gate wait time us"=0, "Record Data Rate"=1, "Count us half of T"=15, "Wait before trigger us"=10100, "Cutoff delay usec"=0} ("Parameters 4"), 10:w92, 11:"PCwriter" ("writer name")) -> (0:w90:errorcluster, 3:w89:refnum<k21>)  [unwired: 2 in]
  n42 = Create Network Stream Reader Endpoint(7:"Data buffer size", 9:fxp<+/-,17,5> 0.0, 10:w85, 11:"PCreaderV" ("reader name")) -> (0:w82:errorcluster, 3:w70:refnum<k21>)  [unwired: 3 in]
  n43 = Create Network Stream Reader Endpoint(7:"Data buffer size", 9:fxp<+/-,17,5> 0.0, 10:w78, 11:"PCreaderI" ("reader name")) -> (0:w75:errorcluster, 3:w73:refnum<k21>)  [unwired: 3 in]
  n44 = Merge Errors(w90, w82, w75) -> (w88:errorcluster)
  n45 = for {
    tunnel: w89 -> [w214]
    tunnel: [w203] -> w71
    tunnel: w88 -> [w144]
    tunnel: [w171] -> w68
    tunnel: w73 -> [w208]
    tunnel: [w206] -> w72
    tunnel: w70 -> [w192]
    tunnel: [w191] -> w69
    tunnel: w40 -> [w177]
    tunnel: w39 -> [w169]
    tunnel: w26 -> [w142] mode=indexing
    i -> [w138]
    stop <- "Stop loop" stop-if-true
    w155 = FALSE ("transpose? (no:F)")
    n46 = Equal?(x=0, y=w138) -> (x = y?=w136:bool)
    n47 = case shown="False" w136 {
      tunnel: [FALSE ("Init") TRUE ("Init")] -> w135
      frame False {
      }
      frame True {
      }
    }
    n48 = call "set single axis Field Module.vi"("Field Device Select"="Field Device Select", "Field sub select"="Field sub select", "error in (no error)"=w144, "Power dbm"="Power dbm", "Init"=w135, "Field Target mT or dBm"=w142, "Exec"=TRUE, "Field Rate mT per sec"="Field Rate mT per sec", "final"=FALSE) -> ("error out"=w143:errorcluster)  [unwired: 10 in]
    n49 = while {
      tunnel: w214 -> [w267]
      tunnel: w143 -> [w266]
      tunnel: [w262] -> w215
      tunnel: [w261] -> w213
      stop <- w263 stop-if-true
      n50 = property class="Network Stream Endpoint"(reference=w267, error in=w266) -> (reference out=w262:refnum<k21>, error out=w261:errorcluster, "AvailElmntsForWrite"=w265:i32)
      n51 = Equal?(x=w265, y=1) -> (x = y?=w263:bool)
    }
    n52 = local read "IV parameters"() -> (w197:T2)
    n53 = Unbundle By Name(w197) -> ("Records Num"=w196:i32, "Record Samples"=w195:u32)
    n54 = To Long Integer(number=w195) -> (32bit integer=w194:i32)
    n55 = Multiply(x=w196, y=w194) -> (x*y=w193:i32)
    n56 = shared-variable-write(w215, w213, w197) -> (w211:refnum<k21>, w212:errorcluster)  [unwired: 1 in, 1 out]
    n57 = for {
      N: w193 -> [_]
      tunnel: w208 -> [w260]
      tunnel: w212 -> [w253]
      tunnel: [w259] -> w176 mode=indexing
      tunnel: [w258] -> _
      tunnel: [w257] -> w190
      tunnel: w192 -> [w256]
      tunnel: [w255] -> w191
      tunnel: [w254] -> w175 mode=indexing
      tunnel: [w252] -> w189
      n58 = call "network stream read.vi"("error in (no error)"=w253, "endpoint in"=w260) -> ("error out"=w257:errorcluster, "Data"=w259:fxp<+/-,17,5>, "endpoint out"=w258:refnum<k21>)  [unwired: 7 in]
      n59 = call "network stream read.vi"("error in (no error)"=w253, "endpoint in"=w256) -> ("error out"=w252:errorcluster, "Data"=w254:fxp<+/-,17,5>, "endpoint out"=w255:refnum<k21>)  [unwired: 7 in]
    }
    n60 = To Double Precision Float(number=w176) -> (double precision float=w154:dbl[])
    n61 = Merge Errors(w190, w189) -> (w182:errorcluster)
    n62 = To Double Precision Float(number=w175) -> (double precision float=w151:dbl[])
    n63 = Multiply(x=w151, y="Voltage Scale factor") -> (x*y=w149:dbl[])
    n64 = Multiply(x=w154, y="Current Scale factor") -> (x*y=w152:dbl[])
    n65 = call "Convert to Dynamic Data2"("Array"=w149) -> ("Dynamic Data Type"=w201:dynamicdata)  [unwired: 3 in]
    n66 = call "Convert to Dynamic Data"("Array"=w152) -> ("Dynamic Data Type"=w202:dynamicdata)  [unwired: 3 in]
    n67 = Array Subset(array=w151, index=0, length="Zero avg") -> (w166:dbl[])
    n68 = To Double Precision Float(number="Zero avg") -> (double precision float=w163:dbl)
    n69 = Add Array Elements(numeric array=w166) -> (sum=w165:dbl)
    n70 = call "Build XY Graph"("Y Input"=w201, "X Input"=w202) -> ("XY Graph"=→"IV curve":cluster{"X":dbl[], "Y":dbl[]}[])  [unwired: 8 in, 1 out]
    n71 = call-poly <vilib>:"Write Delimited Spreadsheet.vi"("file path (dialog if empty)"=w177, "format (%.3f)"="%e", "1D data"=w152, "append to file? (new file:F)"=TRUE, "error in (no error)"=w182, "transpose? (no:F)"=w155) -> ("new file path (Not A Path if cancelled)"=w178:path, "error out"=w179:errorcluster)  [unwired: 8 in]
    n72 = Divide(x=w165, y=w163) -> (x/y=w162:dbl)
    n73 = Add(x=w162, y="Relative threshold") -> (x+y=w145:dbl)
    "Threshold" <- w145
    n74 = call-poly <vilib>:"Write Delimited Spreadsheet.vi"("file path (dialog if empty)"=w178, "format (%.3f)"="%e", "1D data"=w149, "append to file? (new file:F)"=TRUE, "error in (no error)"=w179, "transpose? (no:F)"=w155) -> ("error out"=w158:errorcluster)  [unwired: 8 in, 1 out]
    n75 = To Fixed-Point(fixed-point type=fxp<+,16,4> 0.0 ("AI Trigger Configuration.Hystesis Value"), number=w145) -> (fixed-point=w160:fxp<+,16,4>)
    n76 = flat-sequence {
      tunnel: w160 -> [w222]
      tunnel: w158 -> [w223]
      tunnel: [w223] -> w140
      tunnel: [w227] -> w157
      tunnel: w140 -> [w227]
      tunnel: [w226] -> w139
      frame #0 {
        n77 = Multiply(x=w222, y=fxp<+,16,4> 0.0) -> (x*y=w220:fxp<+,32,8>)
        n78 = local read "Ic parameters"() -> (w225:T2)
        n79 = To Fixed-Point(fixed-point type=fxp<+,16,4> 0.0 ("AI Trigger Configuration.Hystesis Value"), number=w220) -> (fixed-point=w221:fxp<+,16,4>)
        n80 = Bundle By Name(cluster=w225, "AI Trigger Configuration.Trigger Level"=w222, "AI Trigger Configuration.Hystesis Value"=w221) -> (w224:T2)
        n81 = local write "Ic parameters"(w224) -> ()
      }
      frame #1 {
        n82 = local read "Ic parameters"() -> (w226:T2)
      }
    }
    n83 = Unbundle By Name(w139) -> ("Records Num"=w200:i32, "Record Samples"=w199:u32)
    n84 = while {
      tunnel: w211 -> [w249]
      tunnel: w157 -> [w248]
      tunnel: [w246] -> w210
      tunnel: [w245] -> w209
      stop <- w247 stop-if-true
      n85 = property class="Network Stream Endpoint"(reference=w249, error in=w248) -> (reference out=w246:refnum<k21>, error out=w245:errorcluster, "AvailElmntsForWrite"=w251:i32)
      n86 = Equal?(x=w251, y=1) -> (x = y?=w247:bool)
    }
    n87 = To Long Integer(number=w199) -> (32bit integer=w186:i32)
    n88 = Multiply(x=w200, y=w186) -> (x*y=w198:i32)
    n89 = shared-variable-write(w210, w209, w139) -> (w203:refnum<k21>, w207:errorcluster)  [unwired: 1 in, 1 out]
    n90 = for {
      N: w198 -> [_]
      tunnel: w208 -> [w244]
      tunnel: w207 -> [w243]
      tunnel: [w242] -> w172
      tunnel: [w241] -> w206
      tunnel: [w240] -> w204 mode=indexing
      n91 = call "network stream read.vi"("error in (no error)"=w243, "endpoint in"=w244) -> ("error out"=w242:errorcluster, "Data"=w240:fxp<+/-,17,5>, "endpoint out"=w241:refnum<k21>)  [unwired: 7 in]
    }
    n92 = To Double Precision Float(number=w204) -> (double precision float=w170:dbl[])
    n93 = for {
      tunnel: w170 -> [w229] mode=indexing
      tunnel: w186 -> [w235]
      shift-right: [w231] -> w148
      shift-left: dbl[] [] -> [w230]
      i -> [w234]
      n94 = Quotient & Remainder(x=w234, y=w235) -> (x-y*floor(x/y)=w233:i32)  [unwired: 1 out]
      n95 = Equal?(x=1, y=w233) -> (x = y?=w228:bool)
      n96 = case shown="False" w228 {
        tunnel: [w236 w239] -> w231
        tunnel: w230 -> [w236 w238]
        tunnel: w229 -> [_ w237]
        frame False {
        }
        frame True {
          n97 = Build Array (concatenate)(w238, w237) -> (w239:dbl[])
        }
      }
    }
    n98 = local read "Current Scale factor"() -> (w146:dbl)
    n99 = Multiply(x=w148, y=w146) -> (x*y=w147:dbl[])
    n100 = call <vilib>:"Histogram.vi"("intervals"=100, "X"=w147) -> ("Histogram Graph"=→"Histogram Graph":T3)  [unwired: 6 in, 3 out]
    n101 = call-poly <vilib>:"Write Delimited Spreadsheet.vi"("file path (dialog if empty)"=w169, "format (%.3f)"="%e", "1D data"=w147, "append to file? (new file:F)"=TRUE, "error in (no error)"=w172, "transpose? (no:F)"=FALSE) -> ("error out"=w171:errorcluster)  [unwired: 8 in, 1 out]
    "Current Field mT" <- w142
  }
  n102 = local read "Field Device Select"() -> (w10:string)
  n103 = Equal?(x=w10, y="E8257D SG") -> (x = y?=w8:bool)
  n104 = case shown="False" w8 {
    tunnel: [0.0 ("Field Target mT") -135.0 ("Field Target mT")] -> w7
    frame False {
    }
    frame True {
    }
  }
  n105 = Destroy Stream Endpoint(8:w68, 11:w71) -> (0:w81:errorcluster)
  n106 = Destroy Stream Endpoint(8:w81, 11:w72) -> (0:w74:errorcluster)
  n107 = Destroy Stream Endpoint(8:w74, 11:w69) -> (0:w23:errorcluster)
  n108 = call "set single axis Field Module.vi"("Field Device Select"=w10, "error in (no error)"=w23, "Init"=FALSE, "Field Target mT or dBm"=w7, "Exec"=w19, "Field Rate mT per sec"=1.0, "final"=w19) -> ("error out"=w22:errorcluster)  [unwired: 12 in]
  n109 = shared-variable "NI-cRIO-9063\\network varibles.lvlib\\RT Stop"(TRUE ("RT Stop"), error in=w22) -> (error out=w12:errorcluster)
  n110 = call "Stop cRIO fast measure.vi"("error in (no error)"=w12, "VI reference"=w13, "application reference"=w14) -> ("error out"=→"error out":errorcluster)  [unwired: 8 in]
